vi "TopLeft position.vi"(1 "index":i32) -> (0 "TopLeft":T1)   [LabVIEW 2013]
uses:
  <vilib>/Utility/miscctls.llb/LVRowAndColumnUnsignedTypeDef.ctl
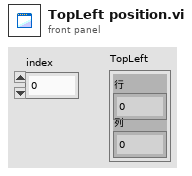
[diagram p1: front panel]
types:
  T1 = typedef "LVRowAndColumnUnsignedTypeDef.ctl" = cluster{"Row":u32, "Column":u32}
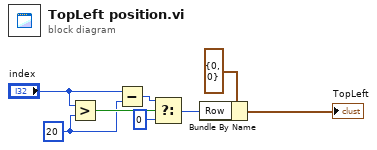
[diagram p0: block diagram]
diagram:
  w4 = 20 ("y")
  n1 = Greater?(x="index", y=w4) -> (0:w6:bool)
  n2 = Subtract(x="index", y=w4) -> (x-y=w3:i32)
  n3 = Select(t=w3, s=w6, f=0) -> (s? t:f=w1:i32)
  n4 = Bundle By Name(cluster=T1 {"Row"=0, "Column"=0} ("左上可见单元格"), "Row"=w1) -> (→"TopLeft":T1)
